vi "Representative_Delta_Position.vi"() -> (0 "New Values In":string[][](array[string])=[["Test data5"]], 1 "New Chs In":string[](array[string])=["30-10-03:New:Channel new5"])   [LabVIEW 2021]
uses:
  Data plotting/subVIs/Plot_Values_Global.vi
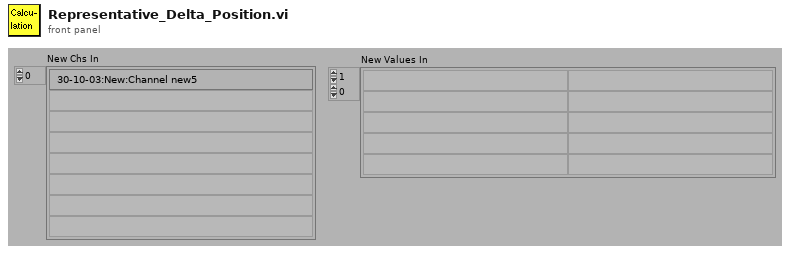
[diagram p1: front panel]
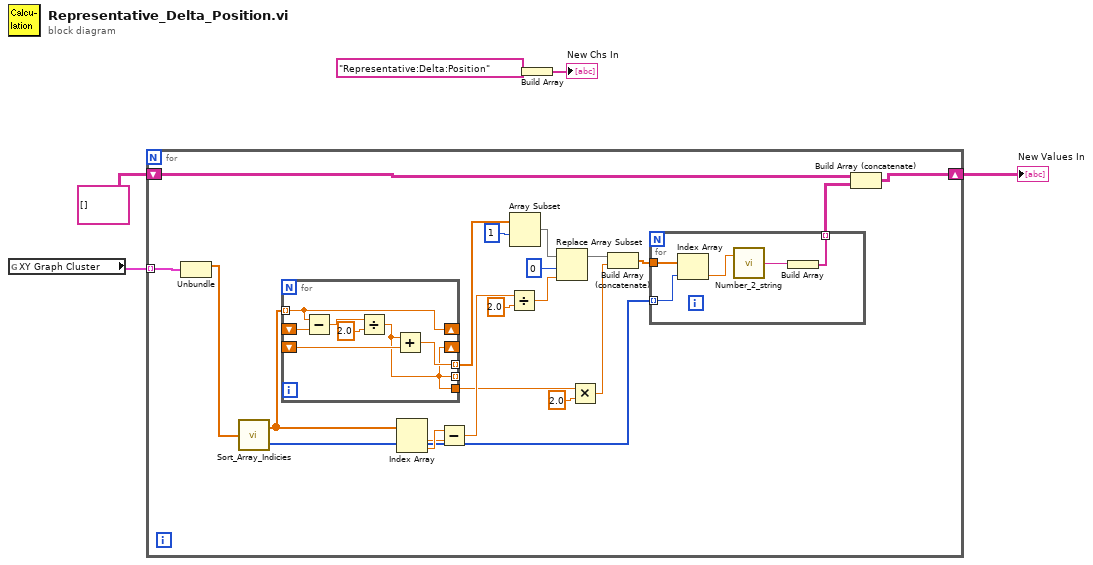
[diagram p0: block diagram]
diagram:
  n1 = global read "Plot_Values_Global.vi" "XY Graph Cluster"() -> (w1:cluster{dbl[], dbl[]}[])
  n2 = for {
    tunnel: w1 -> [w26] mode=indexing
    shift-right: [w24] -> w3
    shift-left: string[][] [] -> [w25]
    n3 = Unbundle(w26) -> (w7:dbl[])  [unwired: 1 out]
    n4 = call "Sort_Array_Indicies.vi"("unsorted array"=w7) -> ("sorted array"=w21:dbl[], "Sort Index"=w9:i32[])
    n5 = for {
      shift-right: [w35] -> _
      shift-left: _ -> [w38]
      tunnel: w21 -> [w35] mode=indexing
      tunnel: [w32] -> _ mode=indexing
      shift-right: [w32] -> _
      shift-left: _ -> [w34]
      tunnel: [w33] -> w23 mode=indexing
      tunnel: [w32] -> w13
      n6 = Subtract(x=w35, y=w38) -> (x-y=w37:dbl)
      n7 = Divide(x=w37, y=2.0) -> (x/y=w32:dbl)
      n8 = Add(x=w32, y=w34) -> (x+y=w33:dbl)
    }
    n9 = Index Array(array=w21) -> (element #1=w19:dbl, element #2=w20:dbl)  [unwired: 2 in]
    n10 = Subtract(x=w20, y=w19) -> (x-y=w16:dbl)
    n11 = Divide(x=w16, y=2.0) -> (x/y=w14:dbl)
    n12 = Array Subset(array=w23, index=1) -> (w18:dbl[])  [unwired: 1 in]
    n13 = Replace Array Subset(array=w18, new element=w14, index=0) -> (w11:dbl[])
    n14 = Multiply(x=w13, y=2.0) -> (x*y=w10:dbl)
    n15 = Build Array (concatenate)(w11, w10) -> (w8:dbl[])
    n16 = for {
      tunnel: w9 -> [w31] mode=indexing
      tunnel: w8 -> [w30]
      tunnel: [w27] -> w6 mode=indexing
      n17 = Index Array(array=w30, index=w31) -> (element=w29:dbl)
      n18 = call "Number_2_string.vi"("number"=w29) -> ("String"=w28:string)  [unwired: 1 in]
      n19 = Build Array(w28) -> (w27:string[])
    }
    n20 = Build Array (concatenate)(w25, w6) -> (w24:string[][])
  }
  "New Values In" <- w3
  n21 = Build Array("Representative:Delta:Position" ("string")) -> (→"New Chs In":string[])
